vi "Set and Unlock Stack.vi"(8 "error in (no error)":errorcluster, 10 "Stack":refnum<class "Device.lvclass">[](array[class]), 11 "IP Connection in":refnum<class "IP Connection.lvclass">) -> (0 "error out":errorcluster, 3 "IP Connection out":refnum<class "IP Connection.lvclass">)   [LabVIEW 2011, in "Tinkerforge.lvlib" / "IP Connection.lvclass"]
doc: "This VI sets the stack and unlocks the data access."
uses:
  IP Connection.lvclass
  Device/Device.lvclass
  IP Connection.lvclass/IP Connection.ctl
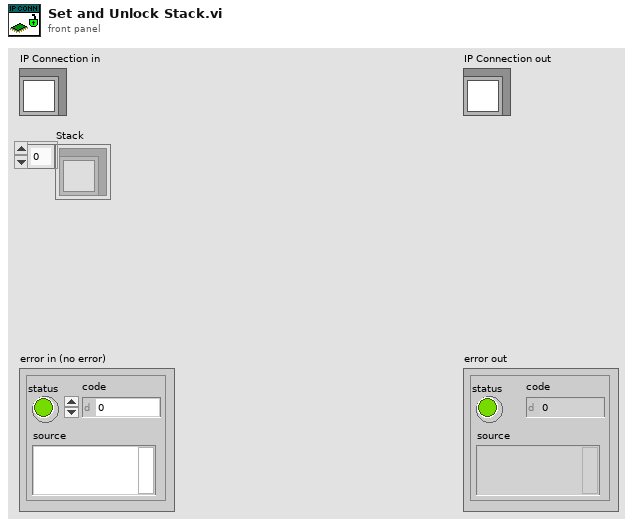
[diagram p1: front panel]
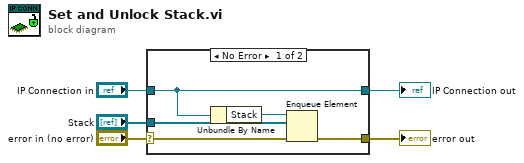
[diagram p0: block diagram]
diagram:
  n1 = case shown="No Error" "error in (no error)" {
    selector: "error in (no error)" -> [w10 w12]
    tunnel: [w9 w12] -> w4
    tunnel: [w8 w11] -> w2
    tunnel: "IP Connection in" -> [w8 w11]
    tunnel: "Stack" -> [w6 _]
    frame No Error {
      n2 = Unbundle By Name(w8) -> ("Stack"=w7:refnum<queue>)
      n3 = Enqueue Element(queue=w7, element=w6, error in (no error)=w10) -> (error out=w9:errorcluster)  [unwired: 1 in, 2 out]
    }
    frame Error {
    }
  }
  "error out" <- w4
  "IP Connection out" <- w2
